vi "NI-DAQmxBaseKernel.vi"() -> (0 "Error Out":errorcluster)   [LabVIEW 2017]
uses:
  Globals/Meas_global.vi
  PWA/PWAtasksGLOBAL.vi
  <vilib>/_DAQmxBase/Internals/DAQmxBase Create Channel (AI-Voltage-Basic).vi
  <vilib>/_DAQmxBase/Internals/DAQmxBase Timing (Sample Clock).vi
  <vilib>/_DAQmxBase/Internals/DAQmxBase Read (Analog 2D DBL NChan NSamp).vi
panel:
  out "CurrentBlock":i32
  out "Case":string
  out "Audit Trail":string[](array[string])
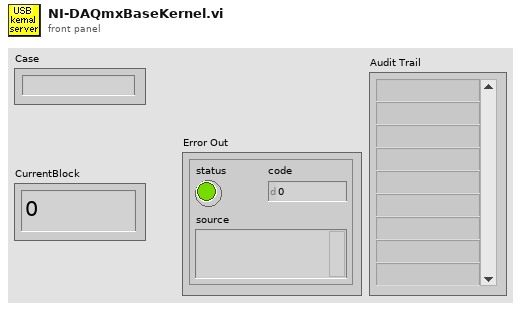
[diagram p1: front panel]
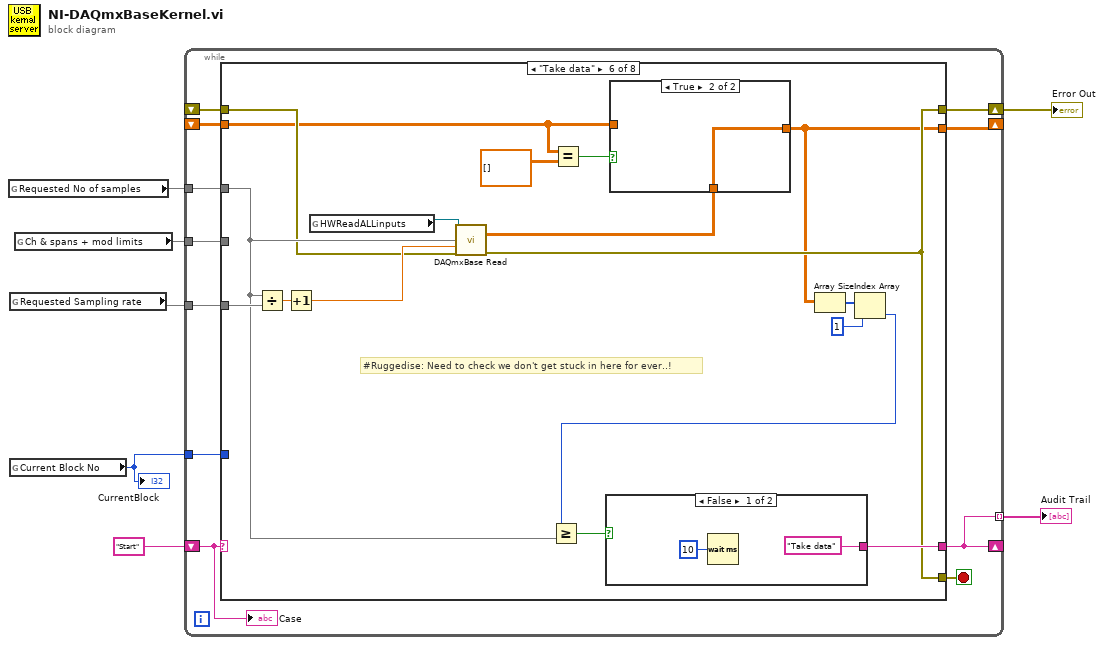
[diagram p0: block diagram]
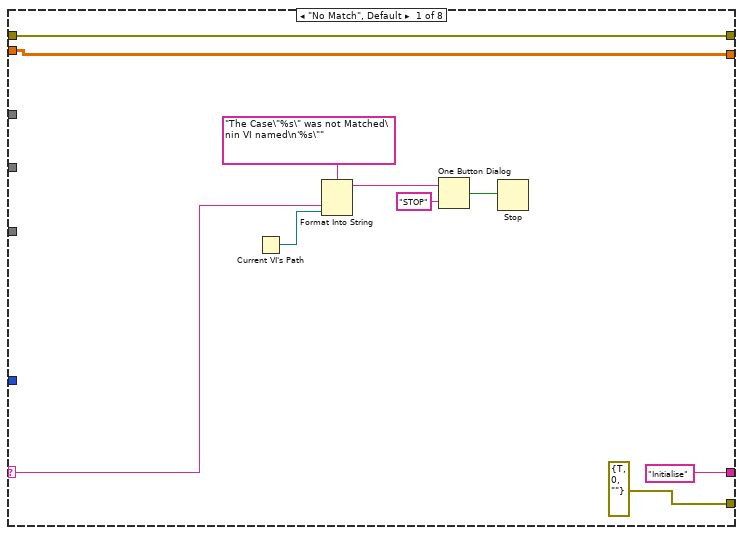
[diagram p2: hidden frame]
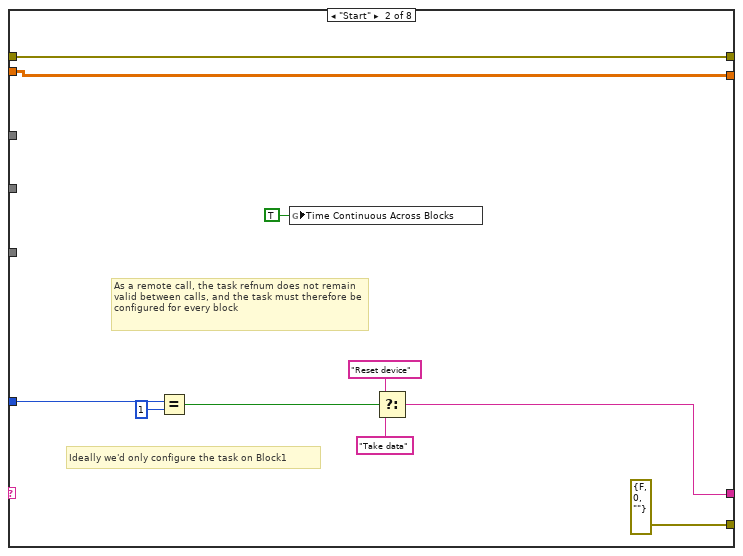
[diagram p3: hidden frame]
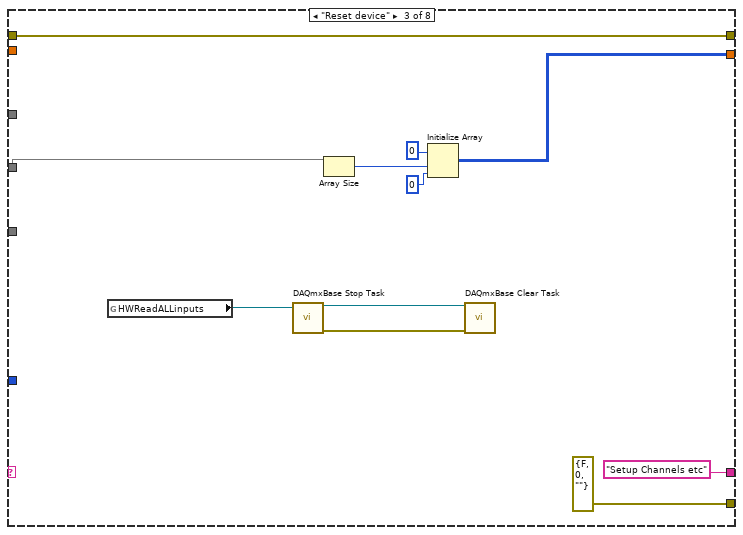
[diagram p4: hidden frame]
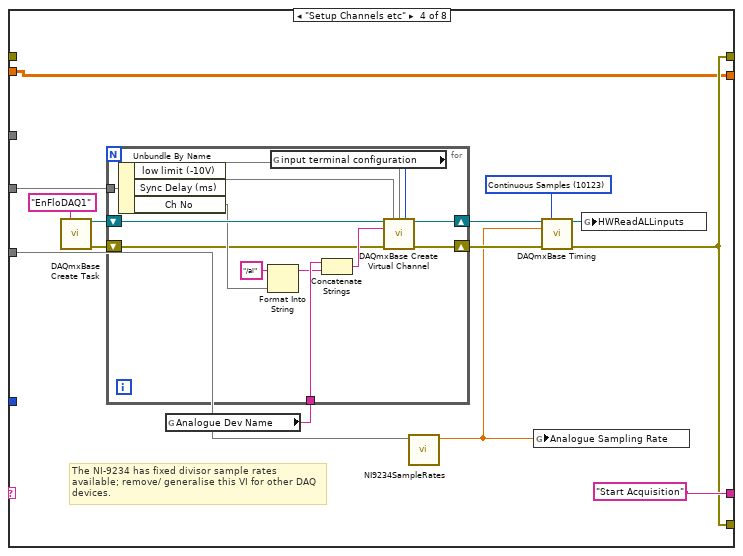
[diagram p5: hidden frame]
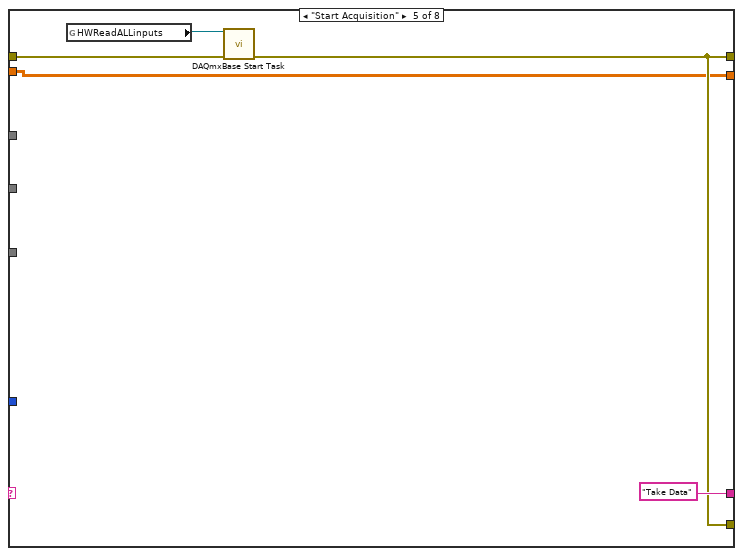
[diagram p6: hidden frame]
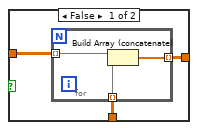
[diagram p7: hidden frame]
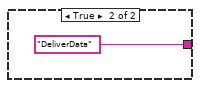
[diagram p8: hidden frame]
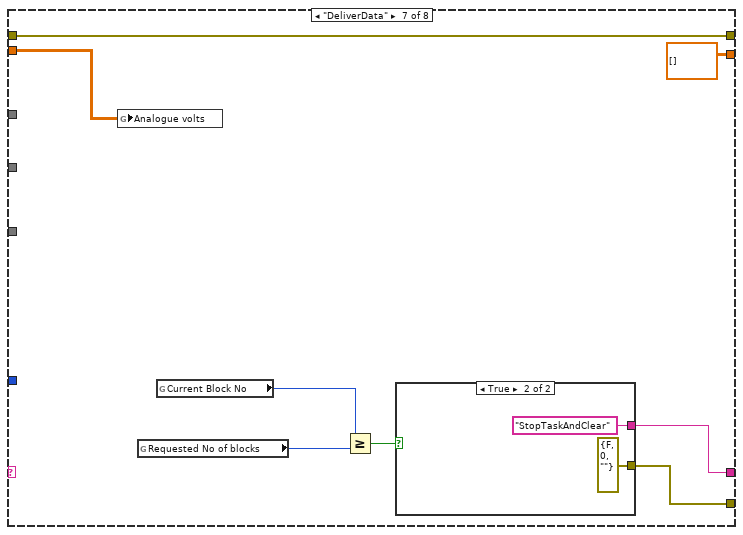
[diagram p9: hidden frame]
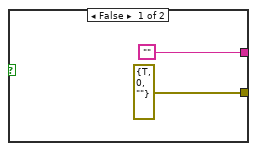
[diagram p10: hidden frame]
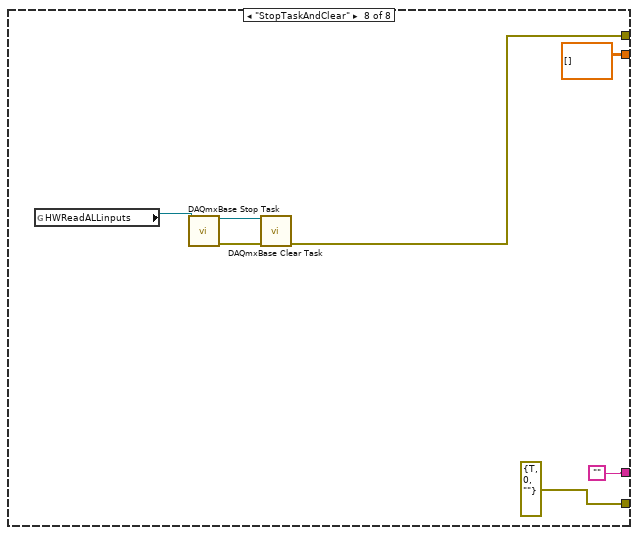
[diagram p11: hidden frame]
diagram:
  n1 = global read "Meas_global.vi" "Requested No of samples"() -> (w5)
  n2 = global read "Meas_global.vi" "Requested Sampling rate"() -> (w6)
  n3 = global read "Meas_global.vi" "Current Block No"() -> (w1:i32)
  "CurrentBlock" <- w1
  n4 = global read "Meas_global.vi" "Ch & spans + mod limits"() -> (w4)
  n5 = while {
    shift-left: "Start" -> [w8]
    shift-right: [w9] -> _
    shift-right: [w17] -> w3
    shift-left: _ -> [w16]
    tunnel: w6 -> [w15]
    tunnel: w5 -> [w14]
    tunnel: w1 -> [w13]
    tunnel: w4 -> [w12]
    shift-right: [w10] -> _
    shift-left: _ -> [w11]
    tunnel: [w9] -> w2 mode=indexing
    stop <- w18 stop-if-true
    n6 = case shown="\"Take data\"" w8 {
      selector: w8 -> [w20 _ _ _ _ _ _ _]
      tunnel: [errorcluster {"status"=TRUE, "code"=0, "source"=""} ("error out") errorcluster {"status"=FALSE, "code"=0, "source"=""} ("error out") errorcluster {"status"=FALSE, "code"=0, "source"=""} ("error out") w55 w79 w92 w113 errorcluster {"status"=TRUE, "code"=0, "source"=""} ("error out")] -> w18
      tunnel: ["Initialise" w36 "Setup Channels etc" "Start Acquisition" "Take Data" w96 w114 ""] -> w9
      tunnel: [w21 w38 w47 w55 w79 w92 w115 w122] -> w17
      tunnel: w16 -> [w21 w38 w47 _ w80 w86 w115 _]
      tunnel: w15 -> [_ _ _ w53 _ w98 _ _]
      tunnel: w14 -> [_ _ _ _ _ w94 _ _]
      tunnel: w13 -> [_ w31 _ _ _ _ _ _]
      tunnel: w12 -> [_ _ w40 w58 _ _ _ _]
      tunnel: w11 -> [w19 w33 _ w54 w78 w83 w116 _]
      tunnel: [w19 w33 w39 w54 w78 w87 dbl[][] [] dbl[][] []] -> w10
      frame "No Match", Default {
        n7 = Current VI's Path() -> (path=w23:path)
        n8 = Format Into String(format string="The Case\"%s\" was not Matched\nin VI named\n'%s\"" ("Format String"), w20, w23) -> (resulting string=w26:string)  [unwired: 2 in, 1 out]
        n9 = One Button Dialog(message=w26, button name ("OK")="STOP") -> (true=w24:bool)
        n10 = Stop(stop? (T)=w24) -> ()
      }
      frame "Start" {
        # "Ideally we'd only configure the task on Block1"
        # "As a remote call, the task refnum does not remain valid between calls, and the task must therefore be configured for every block"
        n11 = Equal?(x=w31, y=1) -> (x = y?=w29:bool)
        n12 = global write "Meas_global.vi" "Time Continuous Across Blocks"(TRUE ("Time Continuous Across Blocks")) -> ()
        n13 = Select(t="Reset device", s=w29, f="Take data") -> (s? t:f=w36:string)
      }
      frame "Reset device" {
        n14 = global read "PWAtasksGLOBAL.vi" "HWReadALLinputs"() -> (w45:refnum<k21>)
        n15 = call <vilib>:"DAQmxBase Stop Task.vi"("task/channels in"=w45) -> ("task out"=w49:refnum<k21>, "error out"=w48:errorcluster)  [unwired: 13 in]
        n16 = Array Size(array=w40) -> (size(s)=w42:i32)
        n17 = Initialize Array(i16 0, w42, 0 ("dimension size")) -> (w39:i16[][])
        n18 = call <vilib>:"DAQmxBase Clear Task.vi"("task in"=w49, "error in"=w48) -> ()  [unwired: 13 in, 1 out]
      }
      frame "Setup Channels etc" {
        w61 = 10123 items=["Finite Samples"=10178, "Continuous Samples"=10123, "Hardware Timed Single Point"=12522] ("sample mode")
        # "The NI-9234 has fixed divisor sample rates available; remove/ generalise this VI for other DAQ devices."
        n19 = call <vilib>:"DAQmxBase Create Task.vi"("new task name"="EnFloDAQ1") -> ("task out"=w59:refnum<k21>, "error out"=w62:errorcluster)  [unwired: 13 in]
        n20 = global read "PWAtasksGLOBAL.vi" "Analogue Dev Name"() -> (w57:string)
        n21 = for {
          tunnel: w58 -> [w76]
          shift-right: [w74] -> w60
          shift-left: w59 -> [w75]
          shift-right: [w73] -> w63
          shift-left: w62 -> [w67]
          tunnel: w57 -> [w72]
          n22 = Unbundle By Name(w76) -> ("low limit (-10V)"=w65, "Sync Delay (ms)"=w64, "Ch No"=w70)
          n23 = Format Into String(initial string="/ai", w70) -> (resulting string=w68:string)  [unwired: 2 in, 1 out]
          n24 = global read "Meas_global.vi" "input terminal configuration"() -> (w66:i32)
          n25 = Concatenate Strings(w72, w68) -> (w71:string)
          n26 = call-poly <vilib>:"DAQmxBase Create Virtual Channel.vi"("task in"=w75, "maximum value"=w64, "minimum value"=w65, "input terminal configuration"=w66, "physical channels"=w71, "error in"=w67) -> ("task out"=w74:refnum<k21>, "error out"=w73:errorcluster)  [unwired: 8 in]
        }
        n27 = call "NI9234SampleRates.vi"("RequestedFrequency(Hz)"=w53) -> ("ClosestHigherFrequency(Hz)"=w52:dbl)  [unwired: 10 in]
        n28 = global write "Meas_global.vi" "Analogue Sampling Rate"(w52) -> ()
        n29 = call-poly <vilib>:"DAQmxBase Timing.vi"("task/channels in"=w60, "sample mode"=w61, "rate"=w52, "error in"=w63) -> ("task out"=w50:refnum<k21>, "error out"=w55:errorcluster)  [unwired: 10 in]
        n30 = global write "PWAtasksGLOBAL.vi" "HWReadALLinputs"(w50) -> ()
      }
      frame "Start Acquisition" {
        n31 = global read "PWAtasksGLOBAL.vi" "HWReadALLinputs"() -> (w77:refnum<k21>)
        n32 = call <vilib>:"DAQmxBase Start Task.vi"("task/channels in"=w77, "error in"=w80) -> ("error out"=w79:errorcluster)  [unwired: 12 in, 1 out]
      }
      frame "Take data" {
        # "#Ruggedise: Need to check we don't get stuck in here for ever..!"
        n33 = Divide(x=w94, y=w98) -> (x/y=w97:dbl)
        n34 = Increment(x=w97) -> (x+1=w93:dbl)
        n35 = global read "PWAtasksGLOBAL.vi" "HWReadALLinputs"() -> (w85:refnum<k21>)
        n36 = call-poly <vilib>:"DAQmxBase Read.vi"("task/channels in"=w85, "number of samples per channel"=w94, "timeout"=w93, "error in"=w86) -> ("data"=w88:dbl[][], "error out"=w92:errorcluster)  [unwired: 9 in, 1 out]
        n37 = Equal?(x=w83, y=dbl[][] []) -> (x = y?=w82:bool)
        n38 = case shown="True" w82 {
          tunnel: w88 -> [w101 w105]
          tunnel: w83 -> [w100 _]
          tunnel: [w99 w105] -> w87
          frame False {
            n39 = for {
              tunnel: w101 -> [w104] mode=indexing
              tunnel: w100 -> [w103] mode=indexing
              tunnel: [w102] -> w99 mode=indexing
              n40 = Build Array (concatenate)(w103, w104) -> (w102:dbl[])
            }
          }
          frame True {
          }
        }
        n41 = Array Size(array=w87) -> (size(s)=w90:i32[])
        n42 = Index Array(array=w90, index=1) -> (element=w89:i32)
        n43 = Greater Or Equal?(x=w89, y=w94) -> (x >= y?=w95:bool)
        n44 = case shown="False" w95 {
          tunnel: ["Take data" "DeliverData"] -> w96
          frame False {
            n45 = Wait (ms)(milliseconds to wait=u32 10) -> ()  [unwired: 1 out]
          }
          frame True {
          }
        }
      }
      frame "DeliverData" {
        n46 = global write "Meas_global.vi" "Analogue volts"(w116) -> ()
        n47 = global read "Meas_global.vi" "Requested No of blocks"() -> (w112:i32)
        n48 = global read "Meas_global.vi" "Current Block No"() -> (w111:i32)
        n49 = Greater Or Equal?(x=w111, y=w112) -> (x >= y?=w110:bool)
        n50 = case shown="True" w110 {
          tunnel: ["" "StopTaskAndClear"] -> w114
          tunnel: [errorcluster {"status"=TRUE, "code"=0, "source"=""} ("error out") errorcluster {"status"=FALSE, "code"=0, "source"=""} ("error out")] -> w113
          frame False {
          }
          frame True {
          }
        }
      }
      frame "StopTaskAndClear" {
        n51 = global read "PWAtasksGLOBAL.vi" "HWReadALLinputs"() -> (w125:refnum<k21>)
        n52 = call <vilib>:"DAQmxBase Stop Task.vi"("task/channels in"=w125) -> ("task out"=w127:refnum<k21>, "error out"=w126:errorcluster)  [unwired: 13 in]
        n53 = call <vilib>:"DAQmxBase Clear Task.vi"("task in"=w127, "error in"=w126) -> ("error out"=w122:errorcluster)  [unwired: 13 in]
      }
    }
    "Case" <- w8
  }
  "Error Out" <- w3
  "Audit Trail" <- w2
